vi "Read Ordered Parameters.vi"(8 "error in (no error)":errorcluster, 10 "TypeMap in":refnum<class "TypeMap.lvclass">, 11 "Object In":variant) -> (0 "error out":errorcluster, 1 "Values":variant[](array[variant]), 2 "Fields":string[](array[string]), 3 "Object Out":variant)   [LabVIEW 2020, in "ORM.lvlib" / "TypeMap.lvclass"]
uses:
  TypeMap.lvclass
  TypeMap.lvclass/TypeMap.ctl
  Read ExplicitFieldOrder.vi
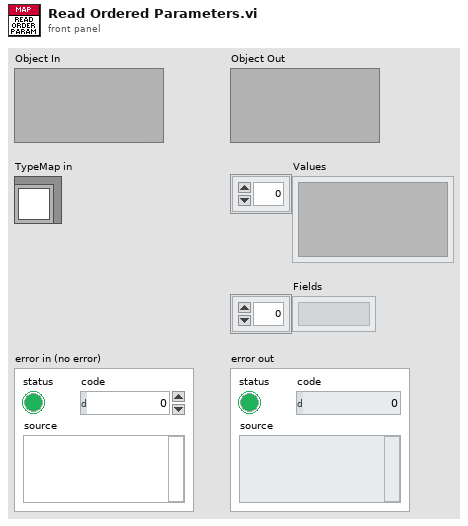
[diagram p1: front panel]
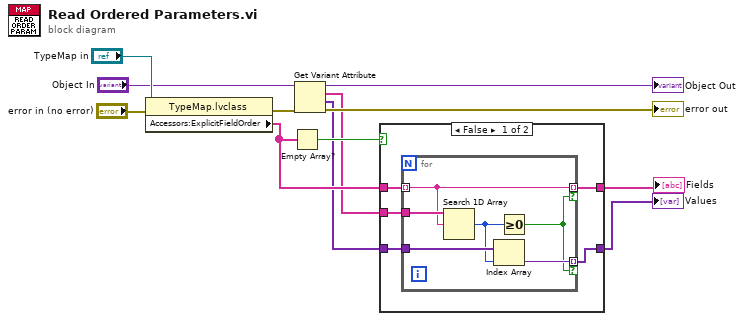
[diagram p0: block diagram]
diagram:
  n1 = property class="TypeMap.lvclass"(reference="TypeMap in", error in="error in (no error)") -> (error out=w12:errorcluster, "Accessors:ExplicitFieldOrder"=w5:string[])  [unwired: 1 out]
  n2 = Empty Array?(array=w5) -> (empty?=w6:bool)
  n3 = Get Variant Attribute(Variant="Object In", error in=w12) -> (duplicate Variant=→"Object Out":variant, names=w4:string[], values=w3:variant[], error out=→"error out":errorcluster)  [unwired: 2 in]
  n4 = case shown="False" w6 {
    tunnel: w5 -> [w17 _]
    tunnel: w4 -> [w16 w25]
    tunnel: w3 -> [w15 w24]
    tunnel: [w14 w25] -> w2
    tunnel: [w13 w24] -> w1
    frame False {
      n5 = for {
        tunnel: w17 -> [w19] mode=indexing
        tunnel: w16 -> [w23]
        tunnel: w15 -> [w22]
        tunnel: [w19] -> w14 mode=indexing if=w20
        tunnel: [w21] -> w13 mode=indexing if=w20
        n6 = Search 1D Array(1D array=w23, element=w19) -> (index of element=w18:i32)  [unwired: 1 in]
        n7 = Index Array(array=w22, index=w18) -> (element=w21:variant)
        n8 = Greater Or Equal To 0?(x=w18) -> (x >= 0?=w20:bool)
      }
    }
    frame True {
    }
  }
  "Fields" <- w2
  "Values" <- w1
